vi "GenEventDisplay.vi"(11 "showAll array":refnum<vi>[](array[refnum])) -> ()   [LabVIEW 2013]
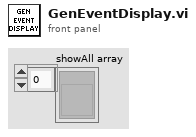
[diagram p1: front panel]
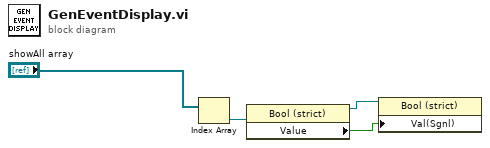
[diagram p0: block diagram]
diagram:
  n1 = Index Array(array="showAll array") -> (element=w2:refnum<vi>)  [unwired: 1 in]
  n2 = property class="Bool (strict)"(reference=w2) -> (reference out=w3:refnum<vi>, "Value"=w4:bool)  [unwired: 1 in, 1 out]
  n3 = property class="Bool (strict)"(reference=w3, "Val(Sgnl)"=w4) -> ()  [unwired: 1 in, 2 out]
